vi "binaryInputs.vi"() -> (3 "inputPort32U":u32)   [LabVIEW 2018]
uses:
  <vilib>/rvi/eio/common/nirviEmuTemplateMethod_errors.vi
  <vilib>/eio/EIONode/EIONode.xnode
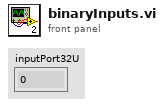
[diagram p1: front panel]
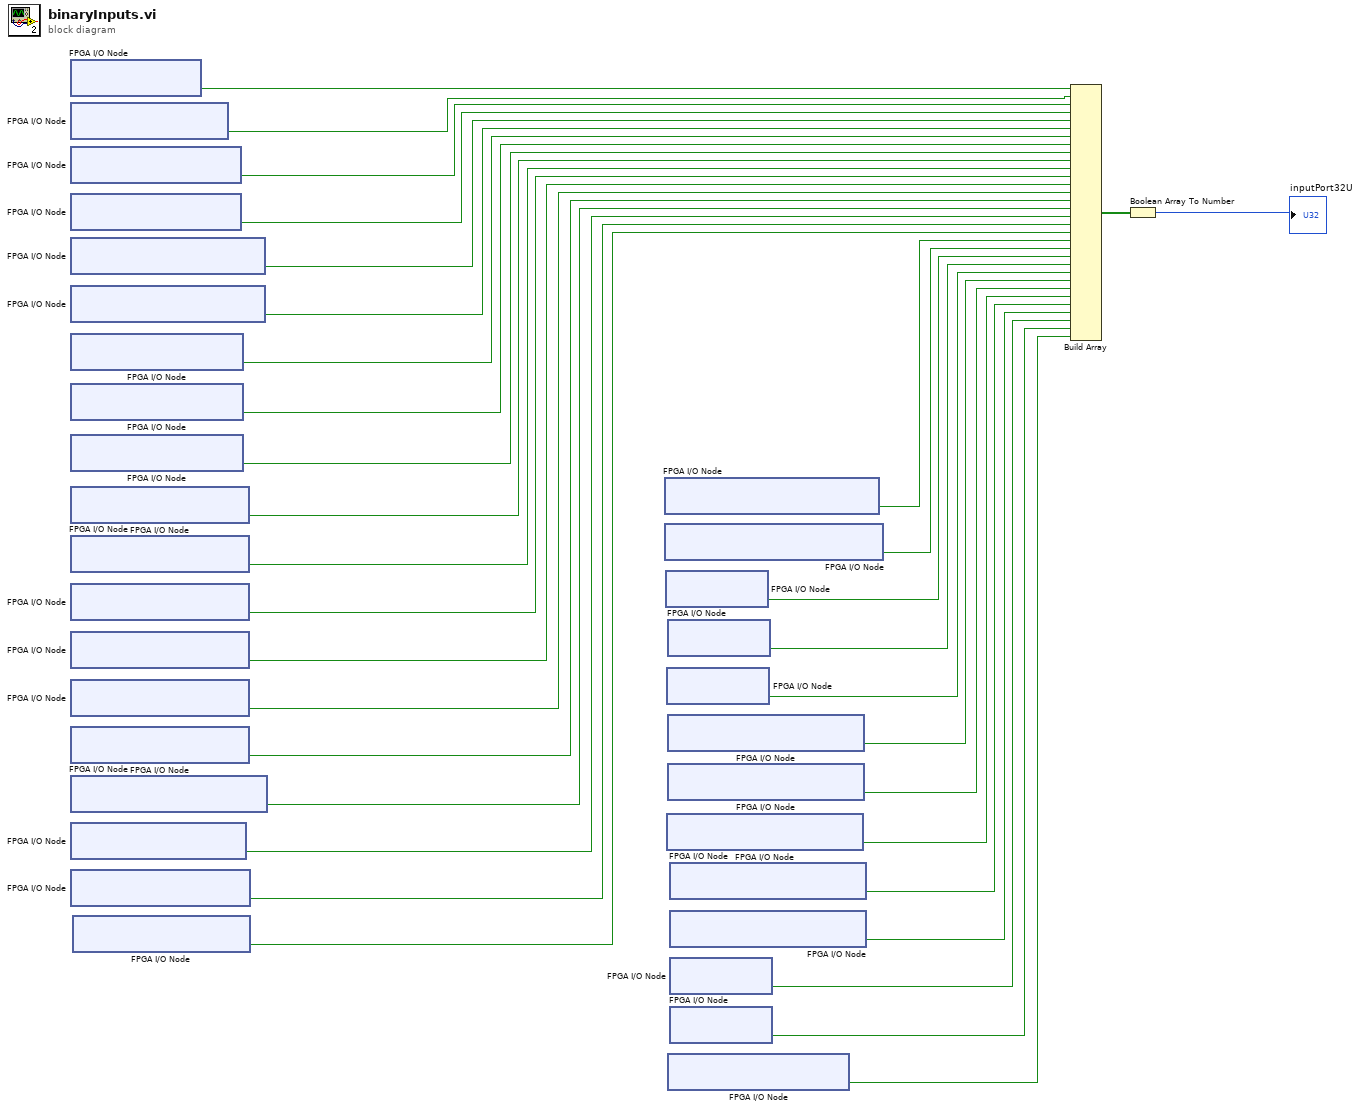
[diagram p0: block diagram]
diagram:
  n1 = xnode "FPGA I/O Node"() -> ("Redundancy_OK"=w2:bool)  [unwired: 1 in, 1 out]
  n2 = xnode "FPGA I/O Node"() -> ("Load_Distribution_OK"=w3:bool)  [unwired: 1 in, 1 out]
  n3 = xnode "FPGA I/O Node"() -> ("Power_Supply_2_DC_OK"=w4:bool)  [unwired: 1 in, 1 out]
  n4 = xnode "FPGA I/O Node"() -> ("Power_Supply_1_DC_OK"=w5:bool)  [unwired: 1 in, 1 out]
  n5 = xnode "FPGA I/O Node"() -> ("Power_Supply_2_Current_OK"=w6:bool)  [unwired: 1 in, 1 out]
  n6 = xnode "FPGA I/O Node"() -> ("Power_Supply_1_Current_OK"=w7:bool)  [unwired: 1 in, 1 out]
  n7 = xnode "FPGA I/O Node"() -> ("J1-W9-1-MtrPwrBrkr_OK"=w8:bool)  [unwired: 1 in, 1 out]
  n8 = xnode "FPGA I/O Node"() -> ("J1-W9-2-MtrPwrBrkr_OK"=w9:bool)  [unwired: 1 in, 1 out]
  n9 = xnode "FPGA I/O Node"() -> ("J1-W9-3-MtrPwrBrkr_OK"=w10:bool)  [unwired: 1 in, 1 out]
  n10 = xnode "FPGA I/O Node"() -> ("J2-W10-1-MtrPwrBrkr_OK"=w11:bool)  [unwired: 1 in, 1 out]
  n11 = xnode "FPGA I/O Node"() -> ("J2-W10-2-MtrPwrBrkr_OK"=w12:bool)  [unwired: 1 in, 1 out]
  n12 = xnode "FPGA I/O Node"() -> ("J2-W10-3-MtrPwrBrkr_OK"=w13:bool)  [unwired: 1 in, 1 out]
  n13 = xnode "FPGA I/O Node"() -> ("J3-W11-1-MtrPwrBrkr_OK"=w14:bool)  [unwired: 1 in, 1 out]
  n14 = xnode "FPGA I/O Node"() -> ("J3-W11-2-MtrPwrBrkr_OK"=w15:bool)  [unwired: 1 in, 1 out]
  n15 = xnode "FPGA I/O Node"() -> ("J3-W11-3-MtrPwrBrkr_OK"=w16:bool)  [unwired: 1 in, 1 out]
  n16 = xnode "FPGA I/O Node"() -> ("J1-W12-1-CommPwrBrkr_OK"=w17:bool)  [unwired: 1 in, 1 out]
  n17 = xnode "FPGA I/O Node"() -> ("ILC_Motor_Power_On_LB"=w18:bool)  [unwired: 1 in, 1 out]
  n18 = xnode "FPGA I/O Node"() -> ("ILC_Comm_Power_On_LB"=w19:bool)  [unwired: 1 in, 1 out]
  n19 = xnode "FPGA I/O Node"() -> ("cRIO_Interlock_Enable_LB"=w20:bool)  [unwired: 1 in, 1 out]
  n20 = xnode "FPGA I/O Node"() -> ("Reset_Motor_Power_Breakers_LB"=w21:bool)  [unwired: 1 in, 1 out]
  n21 = xnode "FPGA I/O Node"() -> ("Reset_Comm_Power_Breakers_LB"=w22:bool)  [unwired: 1 in, 1 out]
  n22 = xnode "FPGA I/O Node"() -> ("Mod5/DI21"=w23:bool)  [unwired: 1 in, 1 out]
  n23 = xnode "FPGA I/O Node"() -> ("Mod5/DI23"=w25:bool)  [unwired: 1 in, 1 out]
  n24 = xnode "FPGA I/O Node"() -> ("J2-W13-2-CommPwrBrkr_OK"=w28:bool)  [unwired: 1 in, 1 out]
  n25 = xnode "FPGA I/O Node"() -> ("Mod5/DI22"=w24:bool)  [unwired: 1 in, 1 out]
  n26 = xnode "FPGA I/O Node"() -> ("J1-W12-2-CommPwrBrkr_OK"=w26:bool)  [unwired: 1 in, 1 out]
  n27 = xnode "FPGA I/O Node"() -> ("J2-W13-1-CommPwrBrkr_OK"=w27:bool)  [unwired: 1 in, 1 out]
  n28 = xnode "FPGA I/O Node"() -> ("Interlock_Power_Relay_On"=w33:bool)  [unwired: 1 in, 1 out]
  n29 = xnode "FPGA I/O Node"() -> ("J3-W14-1-CommPwrBrkr_OK"=w29:bool)  [unwired: 1 in, 1 out]
  n30 = xnode "FPGA I/O Node"() -> ("J3-W14-2-CommPwrBrkr_OK"=w30:bool)  [unwired: 1 in, 1 out]
  n31 = xnode "FPGA I/O Node"() -> ("Mod5/DI29"=w31:bool)  [unwired: 1 in, 1 out]
  n32 = xnode "FPGA I/O Node"() -> ("Mod5/DI30"=w32:bool)  [unwired: 1 in, 1 out]
  n33 = Build Array(w2, w3, w4, w5, w6, w7, w8, w9, w10, w11, w12, w13, w14, w15, w16, w17, w18, w19, w20, w21, w22, w23, w24, w25, w26, w27, w28, w29, w30, w31, w32, w33) -> (w1:bool[])
  n34 = Boolean Array To Number(Boolean array=w1) -> (number=→"inputPort32U":u32)
